vi "LEDseflash.vi"(8 "error in (no error)":errorcluster, 9 "flashspeed":u8, 10 "port":i16, 11 "Id":i16) -> (0 "error out":errorcluster)   [LabVIEW 2015]
uses:
  PacDriveSDK/C#/bin/Debug/PacDrive32.dll
panel:
  out "port(out)":i16
  out "Id(out)":i16
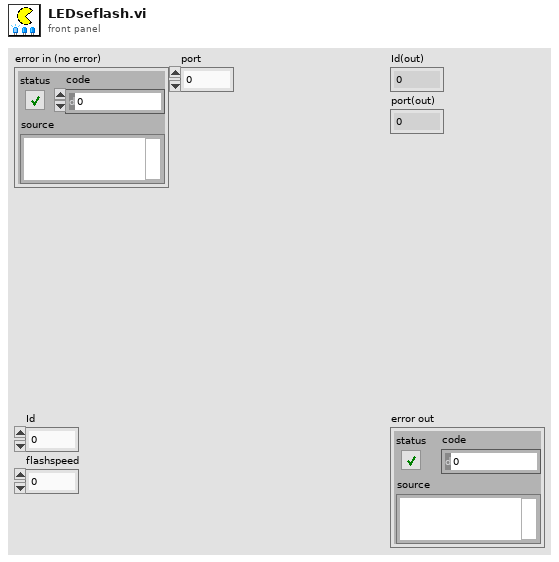
[diagram p1: front panel]
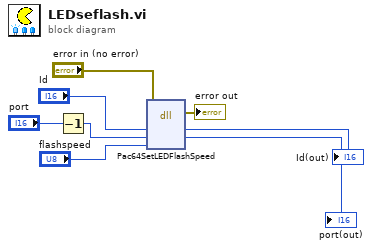
[diagram p0: block diagram]
diagram:
  n1 = Decrement(x="port") -> (x-1=w3:i16)
  n2 = dll-call lib="C:/Users/Team4153/Documents/GitHub/2016_competition/2016 Dashboard Project/TestLights Folder/PacDriveSDK/C#/bin/Debug/PacDrive32.dll" fn="Pac64SetLEDFlashSpeed"(error in="error in (no error)", "Id"="Id", "port"=w3, "flashspeed"="flashspeed") -> (error out=→"error out":errorcluster, "Id"=→"Id(out)":i16, "port"=→"port(out)":i16)  [unwired: 4 in, 1 out]
